vi "Anritsu VNA Convert INT 32 Data Form 1.vi"(8 "Raw Data Point":string) -> (0 "Number":cdb, 1 "Single Array":sgl[](array[numeric]))   [LabVIEW 2011]
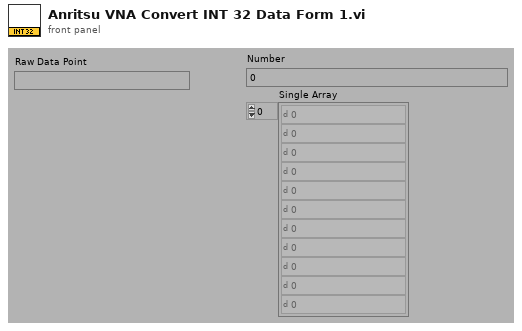
[diagram p1: front panel]
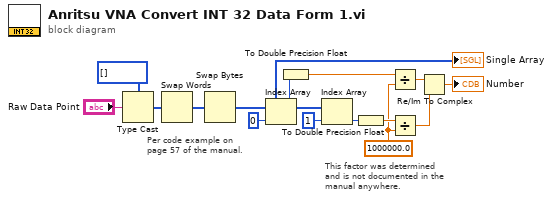
[diagram p0: block diagram]
diagram:
  w3 = 1000000.0 ("y")
  # "This factor was determined\nand is not documented in the\nmanual anywhere."
  # "Per code example on\npage 57 of the manual."
  n1 = Type Cast(type=i32[] [], x="Raw Data Point") -> (*(type *) &x=w7:i32[])
  n2 = Swap Words(1:w7) -> (0:w8:i32[])
  n3 = Swap Bytes(anything=w8) -> (byte swapped=w6:i32[])
  "Single Array" <- w6
  n4 = Index Array(array=w6, index=0) -> (element=w10:i32)
  n5 = To Double Precision Float(number=w10) -> (double precision float=w4:dbl)
  n6 = Index Array(array=w6, index=1) -> (element=w11:i32)
  n7 = To Double Precision Float(number=w11) -> (double precision float=w5:dbl)
  n8 = Divide(x=w4, y=w3) -> (x/y=w2:dbl)
  n9 = Divide(x=w5, y=w3) -> (x/y=w1:dbl)
  n10 = Re/Im To Complex(1:w1, 2:w2) -> (0:→"Number":cdb)
